vi "CalcTimerPeroid.vi"(6 "Exclude Inputs?":bool, 11 "TimePeroid":i32[](array[numeric])) -> (3 "Proper TimePeroid":i32)   [LabVIEW 2017, in "TimerEngine.lvlib" / "TimerEngine.lvclass"]
uses:
  TimerEngine.lvclass
  <userlib>/_OpenG.lib/array/array.llb/Remove Duplicates from 1D Array (I32)__ogtk.vi
  <userlib>/_OpenG.lib/array/array.llb/Filter 1D Array (I32)__ogtk.vi
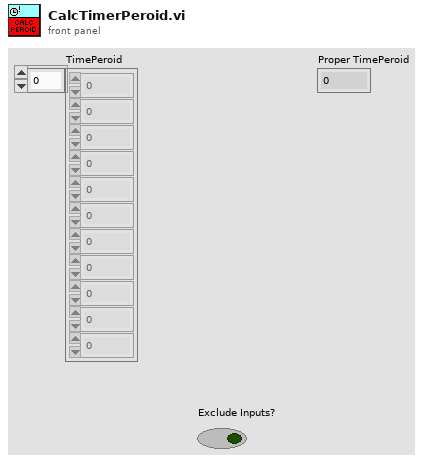
[diagram p1: front panel]
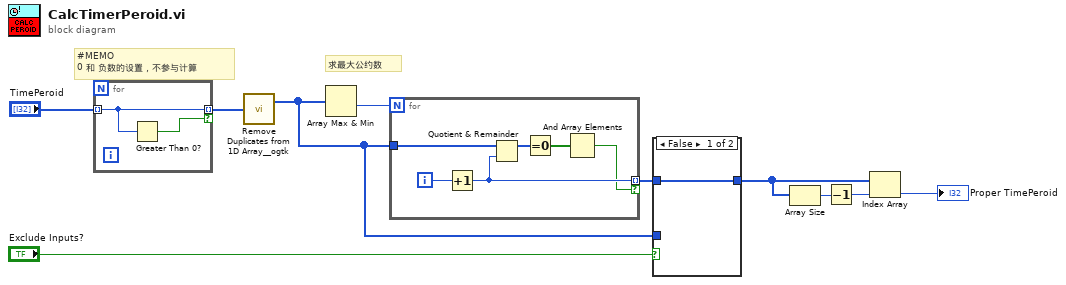
[diagram p0: block diagram]
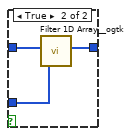
[diagram p2: hidden frame]
diagram:
  # "#MEMO\n0 和 负数的设置，不参与计算"
  # "求最大公约数"
  n1 = for {
    tunnel: "TimePeroid" -> [w12] mode=indexing
    tunnel: [w12] -> w1 mode=indexing if=w11
    n2 = Greater Than 0?(x=w12) -> (x > 0?=w11:bool)
  }
  n3 = call-poly <userlib>:"Remove Duplicates from 1D Array__ogtk.vi"("Input Array"=w1) -> ("Output Array"=w3:i32[])  [unwired: 1 out]
  n4 = Array Max & Min(array=w3) -> (min value=w6:i32)  [unwired: 3 out]
  n5 = for {
    N: w6 -> [_]
    tunnel: [w14] -> w8 mode=indexing if=w13
    tunnel: w3 -> [w16]
    i -> [w17]
    n6 = Increment(x=w17) -> (x+1=w14:i32)
    n7 = Quotient & Remainder(x=w16, y=w14) -> (x-y*floor(x/y)=w18:i32[])  [unwired: 1 out]
    n8 = Equal To 0?(x=w18) -> (x = 0?=w15:bool[])
    n9 = And Array Elements(Boolean array=w15) -> (logical AND=w13:bool)
  }
  n10 = case shown="False" "Exclude Inputs?" {
    tunnel: w8 -> [w19 w22]
    tunnel: [w19 w21] -> w7
    tunnel: w3 -> [_ w20]
    frame False {
    }
    frame True {
      n11 = call-poly <userlib>:"Filter 1D Array__ogtk.vi"("items to filter"=w20, "array"=w22) -> ("filtered array"=w21:i32[])  [unwired: 4 in, 1 out]
    }
  }
  n12 = Array Size(array=w7) -> (size(s)=w10:i32)
  n13 = Decrement(x=w10) -> (x-1=w9:i32)
  n14 = Index Array(array=w7, index=w9) -> (element=→"Proper TimePeroid":i32)
